vi "NMR_Long_RF_Pulse_Sequence_V3.vi"() -> ()   [LabVIEW 2020]
uses:
  <instrlib>/niFgen/niFgen.llb/niFgen Output Mode.ctl
  <instrlib>/niFgen/niFgen.llb/niFgen Waveform Type.ctl
  <instrlib>/niFgen/niFgen.llb/niFgen_ctl Trigger DigEdge - Edge Values (Ring).ctl
  <instrlib>/niFgen/niFgen.llb/niFgen_ctl Trigger Source Values (Ring).ctl
  <instrlib>/niFgen/niFgen.llb/niFgen Trigger Mode.ctl
  <vilib>/Utility/file.llb/Read Delimited Spreadsheet (DBL).vi
  <instrlib>/niFgen/niFgen.llb/niFgen Create Waveform (DBL).vi
  <instrlib>/niFgen/niFgen.llb/niFgen Configure Digital Edge Start Trigger.vi
panel:
  in  "Sample Rate":dbl=12500000.0 format="%.2p"
  in  "FGEN Resource Name 2":refnum<k15>="FGEN2" caption="FGEN Resource Name"
  in  "file to run":path=path "C:/Users/localuser/OneDrive - University of South Carolina/NMR Research/Simulations/wfm.txt"
  in  "Frequency":dbl=27422000.0 format="%.4p"
  in  "Delay Time (ms)":u32=6000
  in  "Number of Scans":i32=1
  in  "Amplitude":dbl=0.35 format="%0_3g"
  in  "FGEN Resource Name":refnum<k15>="Dev1"
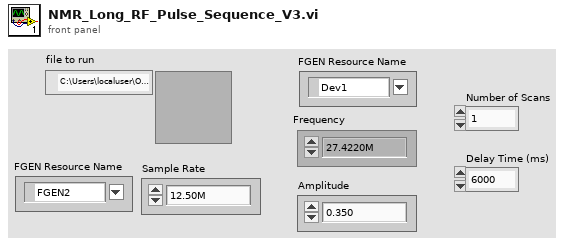
[diagram p1: front panel]
types:
  T1 = typedef "niFgen Output Mode.ctl" = u32
  T2 = typedef "niFgen_ctl Trigger Source Values (Ring).ctl" = string
  T3 = typedef "niFgen Trigger Mode.ctl" = i32
  T4 = typedef "niFgen_ctl Trigger DigEdge - Edge Values (Ring).ctl" = i32
  T5 = typedef "niFgen Waveform Type.ctl" = i32
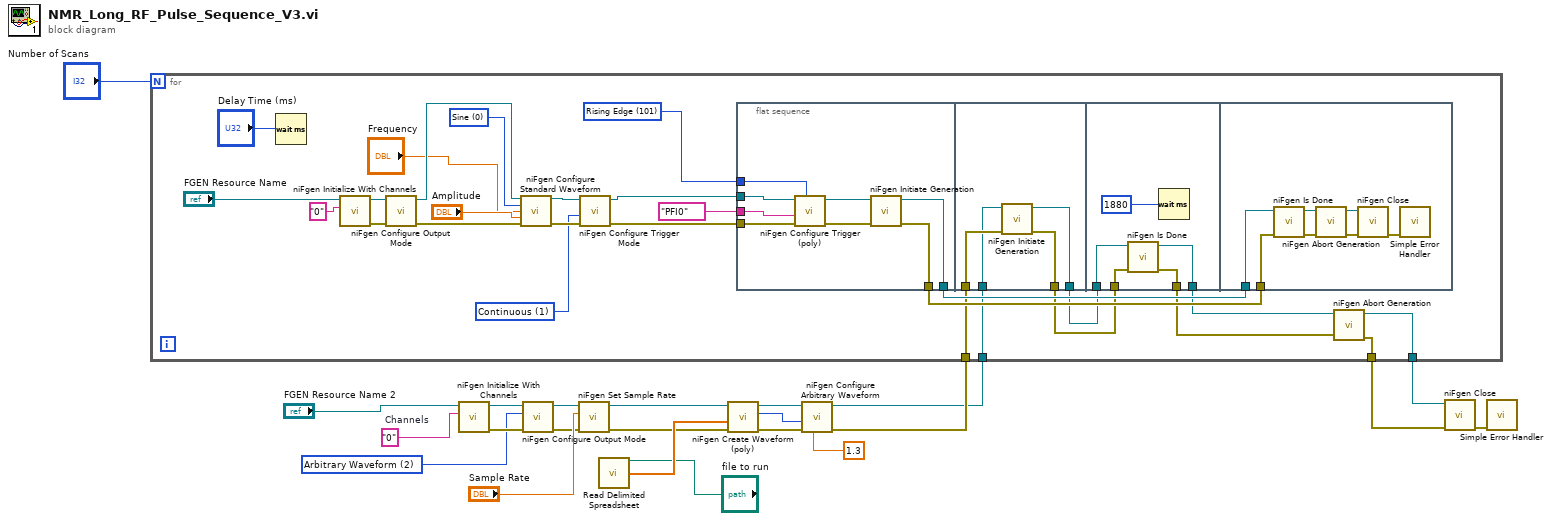
[diagram p0: block diagram]
diagram:
  w7 = "0"  # Channels
  w6 = T1 2 items=["Standard Function", "Frequency List", "Arbitrary Waveform", "Arbitrary Sequence", "Script"] ("output mode")
  n1 = call <instrlib>:"niFgen Initialize With Channels.vi"("Channel Name"=w7, "Resource Name"="FGEN Resource Name 2") -> ("error out"=w10:errorcluster, "Instrument Handle Out"=w11:refnum<k15>)  [unwired: 8 in]
  n2 = call <instrlib>:"niFgen Configure Output Mode.vi"("error in (no error)"=w10, "Output Mode (default: 0=Standard Function)"=w6, "Instrument Handle"=w11) -> ("error out"=w14:errorcluster, "Instrument Handle Out"=w13:refnum<k15>)  [unwired: 6 in]
  n3 = call <instrlib>:"niFgen Set Sample Rate.vi"("error in (no error)"=w14, "Sample Rate (Samp/s)"="Sample Rate", "Instrument Handle"=w13) -> ("error out"=w17:errorcluster, "Instrument Handle Out"=w16:refnum<k15>)  [unwired: 7 in]
  n4 = call-poly <vilib>:"Read Delimited Spreadsheet.vi"("file path (dialog if empty)"="file to run") -> ("first row"=w18:dbl[])  [unwired: 9 in, 5 out]
  n5 = call-poly <instrlib>:"niFgen Create Waveform (poly).vi"("error in (no error)"=w17, "Waveform Data Array"=w18, "Instrument Handle"=w16) -> ("error out"=w20:errorcluster, "Waveform Handle"=w21:i32, "Instrument Handle Out"=w19:refnum<k15>)  [unwired: 6 in]
  n6 = call <instrlib>:"niFgen Configure Arbitrary Waveform.vi"("Gain"=1.3, "error in (no error)"=w20, "Waveform Handle"=w21, "Instrument Handle"=w19) -> ("error out"=w5:errorcluster, "Instrument Handle Out"=w4:refnum<k15>)  [unwired: 6 in]
  n7 = for {
    N: "Number of Scans" -> [_]
    tunnel: w5 -> [w26]
    tunnel: w4 -> [w25]
    tunnel: [w24] -> w2
    tunnel: [w23] -> w1
    w33 = T3 1 items=["Single", "Continuous", "Stepped", "Burst"] ("Trigger Mode (default: 1=continuous)")
    w39 = T4 101 items=["Rising Edge"=101, "Falling Edge"=102] ("Edge (Rising)")
    w41 = T5 0 items=["Sine", "Square", "Triangle", "Ramp Up", "Ramp Down", "DC", "Noise", "User"] ("Waveform")
    n8 = Wait (ms)(milliseconds to wait="Delay Time (ms)") -> ()  [unwired: 1 out]
    n9 = call <instrlib>:"niFgen Initialize With Channels.vi"("Channel Name"="0", "Resource Name"="FGEN Resource Name") -> ("error out"=w46:errorcluster, "Instrument Handle Out"=w49:refnum<k15>)  [unwired: 8 in]
    n10 = call <instrlib>:"niFgen Configure Output Mode.vi"("error in (no error)"=w46, "Instrument Handle"=w49) -> ("error out"=w45:errorcluster, "Instrument Handle Out"=w48:refnum<k15>)  [unwired: 7 in]
    n11 = call <instrlib>:"niFgen Configure Standard Waveform.vi"("Instrument Handle"=w48, "Waveform"=w41, "Frequency"="Frequency", "Amplitude"="Amplitude", "error in (no error)"=w45) -> ("Instrument Handle Out"=w47:refnum<k15>, "error out"=w44:errorcluster)  [unwired: 9 in]
    n12 = call <instrlib>:"niFgen Configure Trigger Mode.vi"("error in (no error)"=w44, "Trigger Mode (default: 1=continuous)"=w33, "Instrument Handle"=w47) -> ("error out"=w38:errorcluster, "Instrument Handle Out"=w36:refnum<k15>)  [unwired: 7 in]
    n13 = flat-sequence {
      tunnel: w39 -> [w56]
      tunnel: w38 -> [w55]
      tunnel: T2 "PFI0" ("Source") -> [w54]
      tunnel: w36 -> [w53]
      tunnel: [w52] -> w34
      tunnel: [w51] -> w35
      tunnel: [w61] -> w31
      tunnel: [w60] -> w30
      tunnel: w26 -> [w59]
      tunnel: w25 -> [w58]
      tunnel: w31 -> [w65]
      tunnel: w30 -> [w64]
      tunnel: [w63] -> w29
      tunnel: [w62] -> w28
      tunnel: w35 -> [w68]
      tunnel: w34 -> [w67]
      frame #0 {
        n14 = call-poly <instrlib>:"niFgen Configure Trigger (poly).vi"("Edge (Rising)"=w56, "error in (no error)"=w55, "Source"=w54, "Instrument Handle"=w53) -> ("error out"=w50:errorcluster, "Instrument Handle Out"=w57:refnum<k15>)  [unwired: 6 in]
        n15 = call <instrlib>:"niFgen Initiate Generation.vi"("error in (no error)"=w50, "Instrument Handle"=w57) -> ("error out"=w51:errorcluster, "Instrument Handle Out"=w52:refnum<k15>)  [unwired: 8 in]
      }
      frame #1 {
        n16 = call <instrlib>:"niFgen Initiate Generation.vi"("error in (no error)"=w59, "Instrument Handle"=w58) -> ("error out"=w61:errorcluster, "Instrument Handle Out"=w60:refnum<k15>)  [unwired: 8 in]
      }
      frame #2 {
        n17 = call <instrlib>:"niFgen Is Done.vi"("error in (no error)"=w65, "Instrument Handle"=w64) -> ("error out"=w63:errorcluster, "Instrument Handle Out"=w62:refnum<k15>)  [unwired: 7 in, 1 out]
        n18 = Wait (ms)(milliseconds to wait=u32 1880) -> ()  [unwired: 1 out]
      }
      frame #3 {
        n19 = call <instrlib>:"niFgen Is Done.vi"("error in (no error)"=w68, "Instrument Handle"=w67) -> ("error out"=w71:errorcluster, "Instrument Handle Out"=w70:refnum<k15>)  [unwired: 7 in, 1 out]
        n20 = call <instrlib>:"niFgen Abort Generation.vi"("error in (no error)"=w71, "Instrument Handle"=w70) -> ("error out"=w72:errorcluster, "Instrument Handle Out"=w73:refnum<k15>)  [unwired: 8 in]
        n21 = call <instrlib>:"niFgen Close.vi"("error in (no error)"=w72, "Instrument Handle"=w73) -> ("error out"=w69:errorcluster)  [unwired: 9 in]
        n22 = call <vilib>:"Simple Error Handler.vi"("error in (no error)"=w69) -> ()  [unwired: 4 in, 5 out]
      }
    }
    n23 = call <instrlib>:"niFgen Abort Generation.vi"("error in (no error)"=w29, "Instrument Handle"=w28) -> ("error out"=w24:errorcluster, "Instrument Handle Out"=w23:refnum<k15>)  [unwired: 8 in]
  }
  n24 = call <instrlib>:"niFgen Close.vi"("error in (no error)"=w2, "Instrument Handle"=w1) -> ("error out"=w3:errorcluster)  [unwired: 9 in]
  n25 = call <vilib>:"Simple Error Handler.vi"("error in (no error)"=w3) -> ()  [unwired: 4 in, 5 out]
